vi "KT2_2.vi"() -> ()   [LabVIEW 2018]
uses:
  Global 5.vi
  Downloads/Global 2.vi
  Global 4.vi
panel:
  out "Waveform Chart":dbl(graph)
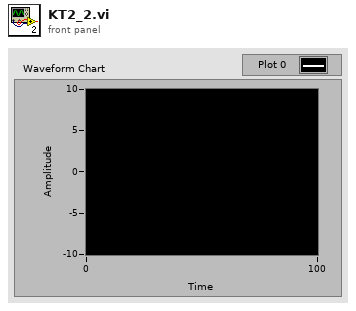
[diagram p1: front panel]
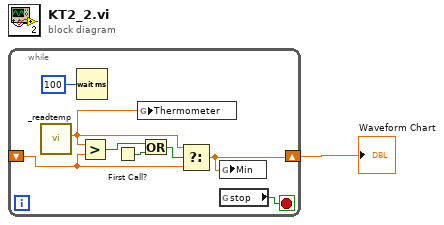
[diagram p0: block diagram]
diagram:
  n1 = while {
    shift-right: [w3] -> w1
    shift-left: _ -> [w8]
    stop <- w4 stop-if-true
    n2 = call "_readtemp.vi"() -> ("Temperature"=w2:dbl)  [unwired: 10 in, 1 out]
    n3 = Wait (ms)(milliseconds to wait=u32 100) -> ()  [unwired: 1 out]
    n4 = Greater?(x=w2, y=w8) -> (0:w5:bool)
    n5 = First Call?() -> (First Call?: T/F=w6:bool)
    n6 = global write "Global 5.vi" "Thermometer"(w2) -> ()
    n7 = Or(x=w5, y=w6) -> (x .or. y?=w9:bool)
    n8 = Select(t=w2, s=w9, f=w8) -> (s? t:f=w3:dbl)
    n9 = global write "Global 4.vi" "Min"(w3) -> ()
    n10 = global read "Global 2.vi" "stop"() -> (w4:bool)
  }
  "Waveform Chart" <- w1
